vi "FGV FT-IR Parameter.vi"(0 "NoOfGasses neu":i32, 1 "NoOfScan neu":u32, 2 "Komm Stoppen":bool, 3 "Einstellungen":T2, 4 "Ausgangs-Cluster":T1, 5 "Spektrum loggen aktiv?":bool, 7 "Aktion":T3) -> (12 "Komm Stoppen":bool, 13 "Ausgangs-Cluster":T1, 14 "Instrument State":string, 15 "NoOfGasses":u32, 16 "Current Recipe":string, 17 "NoOfScan":u32, 18 "Zykluszeit Messdatenverteiler":u32, 19 "Zykluszeit ToolWeb":u32)   [LabVIEW 2020, in "FT-IR.lvlib"]
uses:
  FT-IR.lvlib
  FGV FT-IR Aktionen.ctl
  TOOLweb Interface Library/TOOLweb Einstellungen.ctl
  Aktionen Parameter Laden-Speichern.ctl
  TOOLweb Interface Library/Typdefinitionen.lvlib
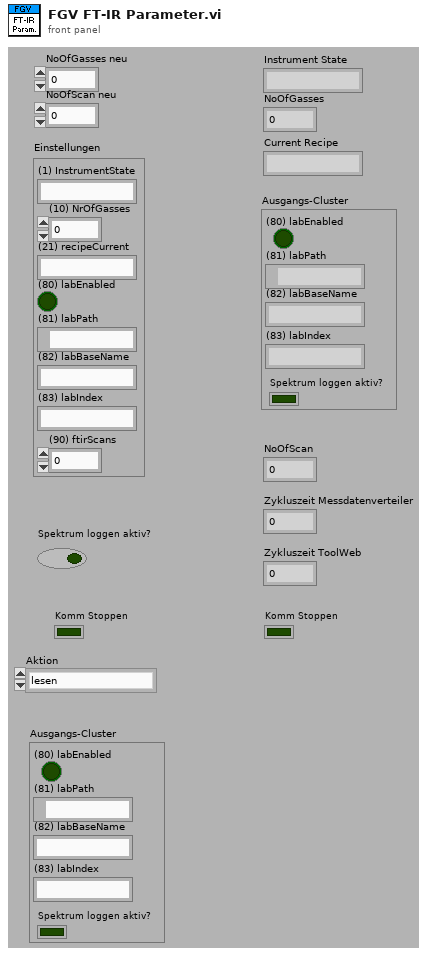
[diagram p1: front panel]
types:
  T1 = cluster{"(80) labEnabled":bool, "(81) labPath":path, "(82) labBaseName":string, "(83) labIndex":string, "Spektrum loggen aktiv?":bool}
  T2 = typedef "FT-IR.lvlib/TOOLweb Interface.lvlib/Typdefinitionen.lvlib/TOOLweb Einstellungen.ctl" = cluster{"(1) InstrumentState":string, "(10) NrOfGasses":i32, "(21) recipeCurrent":string, "(80) labEnabled":bool, "(81) labPath":path, "(82) labBaseName":string, "(83) labIndex":string, "(90) ftirScans":i32}
  T3 = typedef "FT-IR.lvlib/FGV FT-IR Aktionen.ctl" = enum16{"lesen", "NOG setzen", "NOS setzen", "Initialisieren", "speichern", "ALLES setzen", "FT-IR Spektrum loggen", "Komm Stoppen", "Spektrum LogKonfig"}
  T4 = typedef "FT-IR.lvlib/Aktionen Parameter Laden-Speichern.ctl" = enum16{"laden", "speichern"}
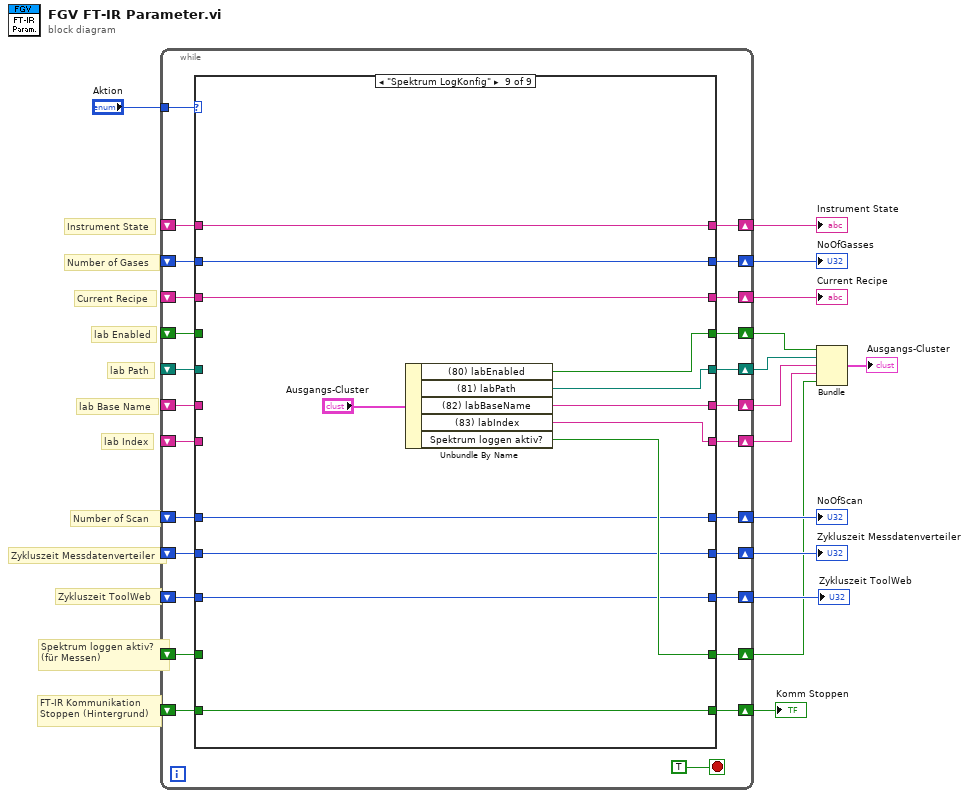
[diagram p0: block diagram]
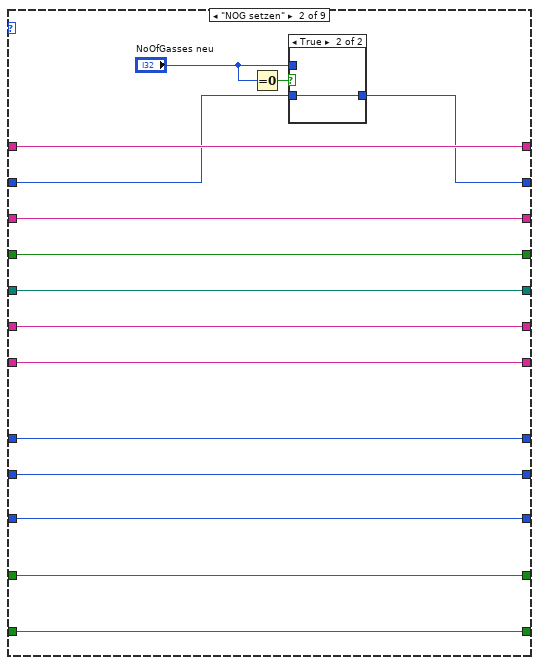
[diagram p3: hidden frame]
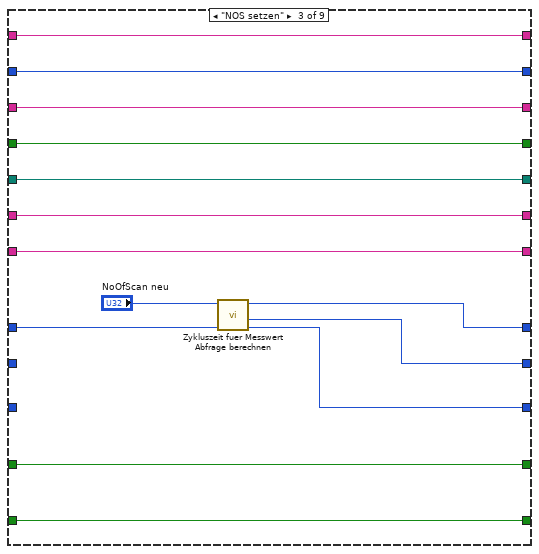
[diagram p5: hidden frame]
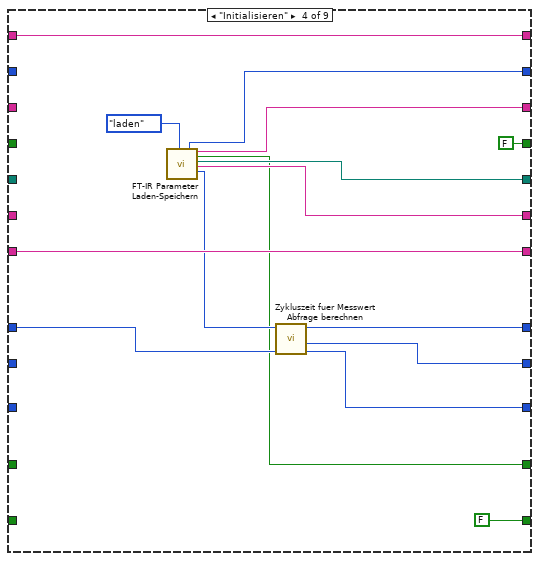
[diagram p6: hidden frame]
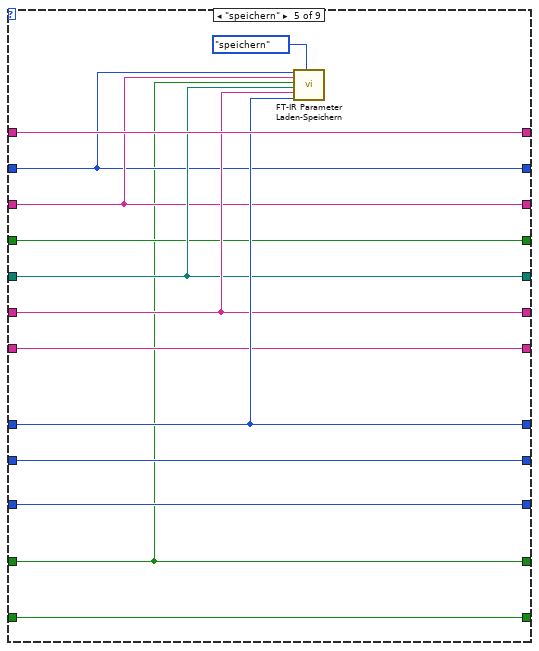
[diagram p7: hidden frame]
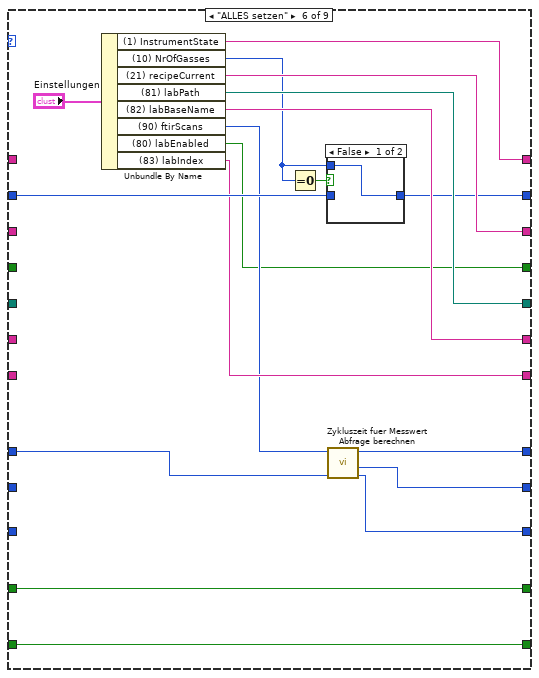
[diagram p8: hidden frame]
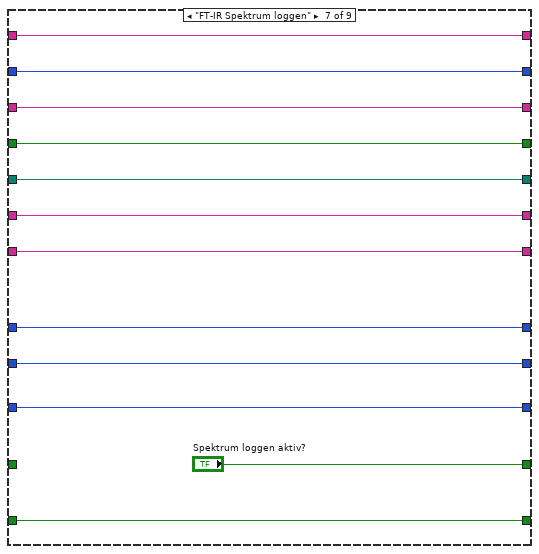
[diagram p10: hidden frame]
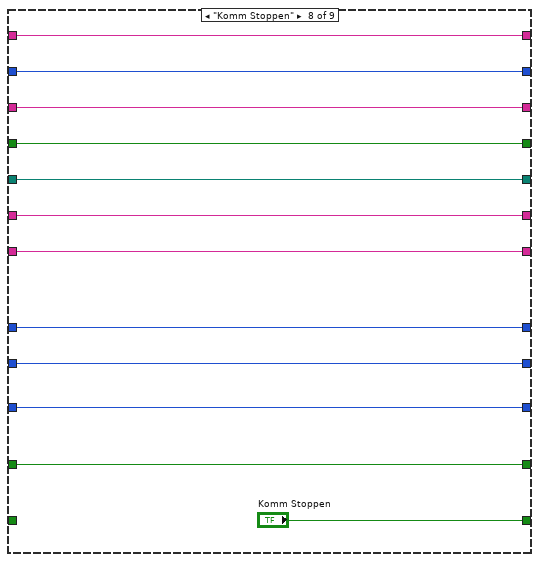
[diagram p11: hidden frame]
diagram:
  # "FT-IR Kommunikation\nStoppen (Hintergrund)"
  # "lab Index"
  # "Zykluszeit ToolWeb"
  # "Spektrum loggen aktiv? \n(für Messen)"
  # "lab Base Name"
  # "lab Path"
  # "lab Enabled"
  # "Current Recipe"
  # "Instrument State"
  # "Zykluszeit Messdatenverteiler"
  # "Number of Scan"
  # "Number of Gases"
  n1 = while {
    shift-right: [w40] -> w9
    shift-left: _ -> [w38]
    tunnel: "Aktion" -> [w39]
    shift-right: [w35] -> w7
    shift-left: _ -> [w36]
    shift-right: [w34] -> w6
    shift-left: _ -> [w33]
    shift-right: [w32] -> w10
    shift-left: _ -> [w31]
    shift-right: [w30] -> w8
    shift-left: _ -> [w29]
    shift-right: [w28] -> w13
    shift-left: _ -> [w25]
    shift-right: [w27] -> w12
    shift-left: _ -> [w24]
    shift-right: [w26] -> w11
    shift-left: _ -> [w23]
    shift-right: [w22] -> w4
    shift-left: _ -> [w21]
    shift-right: [w19] -> w5
    shift-left: _ -> [w20]
    shift-right: [w17] -> w3
    shift-left: _ -> [w18]
    shift-right: [w15] -> w1
    shift-left: _ -> [w16]
    stop <- TRUE stop-if-true
    n2 = case shown="\"Spektrum LogKonfig\"" w39 {
      tunnel: [w52 w58 w83 w97 w104 w121 w136 w155 w161] -> w40
      tunnel: w38 -> [w52 w57 w83 _ w104 w122 w136 w155 w161]
      tunnel: [w51 w67 w73 w90 w109 w117 w141 w154 w159] -> w35
      tunnel: w36 -> [w51 w67 w74 w89 w109 w118 w141 w154 w159]
      tunnel: [w50 w66 w71 w87 w110 w116 w142 w153 w158] -> w34
      tunnel: w33 -> [w50 w66 _ _ w110 _ w142 w153 w158]
      tunnel: [w49 w65 w81 w98 w111 w128 w135 w152 w162] -> w32
      tunnel: w31 -> [w49 w65 w81 w98 w111 _ w135 w152 w162]
      tunnel: [w48 w64 w82 w96 w105 w127 w137 w151 w160] -> w30
      tunnel: w29 -> [w48 w64 w82 _ w105 _ w137 w151 w160]
      tunnel: [w47 w63 w80 FALSE ("(80) labEnabled") w106 w113 w138 w150 w163] -> w28
      tunnel: [w46 w62 w79 w95 w107 w126 w139 w149 w164] -> w27
      tunnel: [w45 w61 w78 w94 w108 w125 w140 w148 w165] -> w26
      tunnel: w25 -> [w47 w63 w80 _ w106 _ w138 w150 _]
      tunnel: w24 -> [w46 w62 w79 _ w107 _ w139 w149 _]
      tunnel: w23 -> [w45 w61 w78 _ w108 _ w140 w148 _]
      tunnel: [w44 w60 w77 w84 w99 w112 "Spektrum loggen aktiv?" w147 w167] -> w22
      tunnel: w21 -> [w44 w60 w77 _ w99 w112 _ w147 _]
      tunnel: w20 -> [w43 w55 _ _ w103 _ w134 w146 w157]
      tunnel: [w43 w55 w72 w88 w103 w115 w134 w146 w157] -> w19
      tunnel: w18 -> [w42 w54 w76 w93 w102 _ w133 w145 _]
      tunnel: [w42 w54 w76 w93 w102 w120 w133 w145 w166] -> w17
      tunnel: w16 -> [w41 w53 w70 _ w100 w114 w132 _ w156]
      tunnel: [w41 w53 w70 FALSE ("Komm Stoppen") w100 w114 w132 "Komm Stoppen" w156] -> w15
      frame "lesen", Default {
      }
      frame "NOG setzen" {
        n3 = Equal To 0?(x="NoOfGasses neu") -> (x = 0?=w59:bool)
        n4 = case shown="True" w59 {
          tunnel: "NoOfGasses neu" -> [w68 _]
          tunnel: w57 -> [_ w69]
          tunnel: [w68 w69] -> w58
          frame False {
          }
          frame True {
          }
        }
      }
      frame "NOS setzen" {
        n5 = call "Zykluszeit fuer Messwert Abfrage berechnen.vi"("NoOfScan ALT"=w74, "NoOfScan NEU"="NoOfScan neu") -> ("Zykluszeit ToolWeb"=w72:u32, "Zykluszeit Messdatenverteiler"=w71:u32, "NoOfScan"=w73:u32)  [unwired: 7 in]
      }
      frame "Initialisieren" {
        n6 = call "FT-IR Parameter Laden-Speichern.vi"("Aktion"=Aktionen_Parameter_Laden-Speichern."laden") -> ("NoOfGases"=w97:u32, "CurrentRecipe"=w96:string, "labEnabled"=w84:bool, "labPath"=w95:path, "labBaseName"=w94:string, "NoOfScan"=w91:u32)  [unwired: 13 in]
        n7 = call "Zykluszeit fuer Messwert Abfrage berechnen.vi"("NoOfScan ALT"=w89, "NoOfScan NEU"=w91) -> ("Zykluszeit ToolWeb"=w88:u32, "Zykluszeit Messdatenverteiler"=w87:u32, "NoOfScan"=w90:u32)  [unwired: 7 in]
      }
      frame "speichern" {
        n8 = call "FT-IR Parameter Laden-Speichern.vi"("NoOfGases In"=w104, "CurrentRecipe In"=w105, "labEnabled In"=w99, "labPath In"=w107, "labBaseName In"=w108, "NoOfScan In"=w109, "Aktion"=Aktionen_Parameter_Laden-Speichern."speichern") -> ()  [unwired: 7 in, 6 out]
      }
      frame "ALLES setzen" {
        n9 = Unbundle By Name("Einstellungen") -> ("(1) InstrumentState"=w128:string, "(10) NrOfGasses"=w123:i32, "(21) recipeCurrent"=w127:string, "(81) labPath"=w126:path, "(82) labBaseName"=w125:string, "(90) ftirScans"=w119:i32, "(80) labEnabled"=w113:bool, "(83) labIndex"=w120:string)
        n10 = Equal To 0?(x=w123) -> (x = 0?=w124:bool)
        n11 = case shown="False" w124 {
          tunnel: w123 -> [w130 _]
          tunnel: w122 -> [_ w131]
          tunnel: [w130 w131] -> w121
          frame False {
          }
          frame True {
          }
        }
        n12 = call "Zykluszeit fuer Messwert Abfrage berechnen.vi"("NoOfScan ALT"=w118, "NoOfScan NEU"=w119) -> ("Zykluszeit ToolWeb"=w115:u32, "Zykluszeit Messdatenverteiler"=w116:u32, "NoOfScan"=w117:u32)  [unwired: 7 in]
      }
      frame "FT-IR Spektrum loggen" {
      }
      frame "Komm Stoppen" {
      }
      frame "Spektrum LogKonfig" {
        n13 = Unbundle By Name("Ausgangs-Cluster") -> ("(80) labEnabled"=w163:bool, "(81) labPath"=w164:path, "(82) labBaseName"=w165:string, "(83) labIndex"=w166:string, "Spektrum loggen aktiv?"=w167:bool)
      }
    }
  }
  "NoOfGasses" <- w9
  "NoOfScan" <- w7
  "Zykluszeit Messdatenverteiler" <- w6
  "Current Recipe" <- w8
  "Instrument State" <- w10
  "Zykluszeit ToolWeb" <- w5
  "Komm Stoppen" <- w1
  n14 = Bundle("(80) labEnabled"=w13, "(81) labPath"=w12, "(82) labBaseName"=w11, "(83) labIndex"=w3, "Spektrum loggen aktiv?"=w4) -> (→"Ausgangs-Cluster":T1)  [unwired: 1 in]
